vi "Move To Impl.vi"(8 "error in (no error)":errorcluster, 9 "Index":u16, 10 "Area":enum16{"Home", "Well", "Wash Port"}(ring), 11 "Simulated Autosampler in":refnum<class "Simulated Autosampler.lvclass">) -> (0 "error out":errorcluster, 3 "Simulated Autosampler out":refnum<class "Simulated Autosampler.lvclass">)   [LabVIEW 2023, in "Simulated Autosampler.lvlib" / "Simulated Autosampler.lvclass"]
uses:
  Simulated Autosampler.lvclass
  Simulated Autosampler.lvclass/Simulated Autosampler.ctl
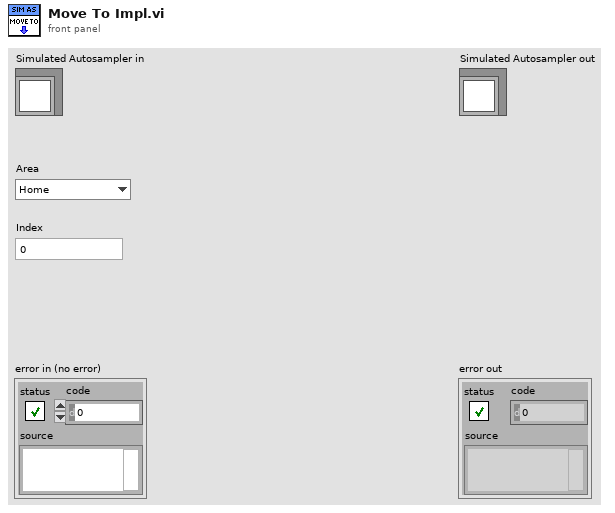
[diagram p1: front panel]
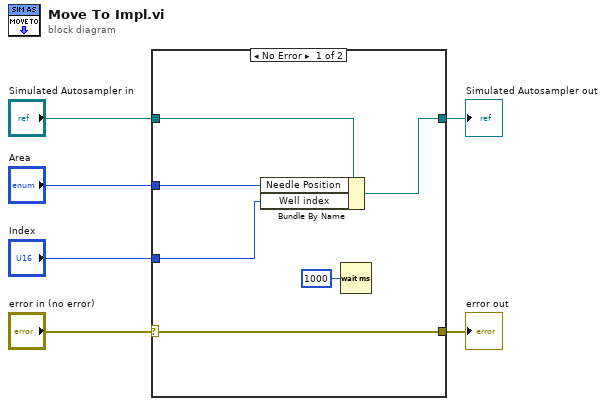
[diagram p0: block diagram]
diagram:
  n1 = case shown="No Error" "error in (no error)" {
    selector: "error in (no error)" -> [w12 w13]
    tunnel: [w12 w13] -> w5
    tunnel: "Simulated Autosampler in" -> [w11 w14]
    tunnel: [w10 w14] -> w3
    tunnel: "Index" -> [w9 _]
    tunnel: "Area" -> [w8 _]
    frame No Error {
      n2 = Bundle By Name(cluster=w11, "Needle Position"=w8, "Well index"=w9) -> (w10:refnum<class "Simulated Autosampler.lvclass">)
      n3 = Wait (ms)(milliseconds to wait=u32 1000) -> ()  [unwired: 1 out]
    }
    frame Error {
    }
  }
  "error out" <- w5
  "Simulated Autosampler out" <- w3
